vi "PVCamGlobalVariables.vi"() -> ()   [LabVIEW 2018]
panel:
  out "Histogram Enabled":bool
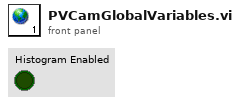
[diagram p1: front panel]
diagram:
